vi "AP2x4x ScaleXUnit.vi"(7 "Unit":enum16{"Frequency", "Wavelength"}(ring), 8 "error in":errorcluster, 11 "AP2x4x IN":refnum<visa-resource-name>="TCPIP0::169.254.53.138::5900::SOCKET") -> (0 "error out":errorcluster, 3 "AP2x4x OUT":refnum<visa-resource-name>="TCPIP0::169.254.53.138::5900::SOCKET")   [LabVIEW 2014]
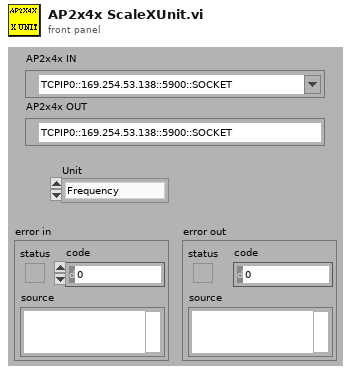
[diagram p1: front panel]
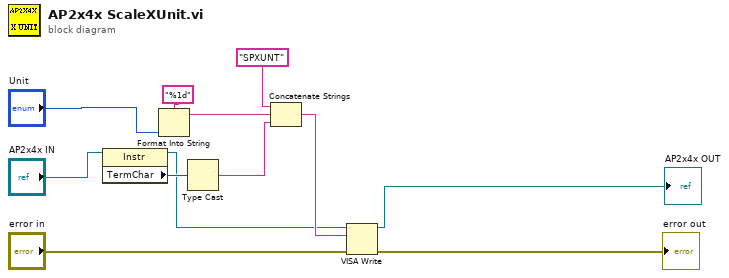
[diagram p0: block diagram]
diagram:
  n1 = property class="Instr"(reference="AP2x4x IN") -> (reference out=w7:refnum<visa-resource-name>, "TermChar"=w10:u8)  [unwired: 1 in, 1 out]
  n2 = Format Into String(format string="%1d", "Unit") -> (resulting string=w5:string)  [unwired: 2 in, 1 out]
  n3 = Type Cast(x=w10) -> (*(type *) &x=w8:string)  [unwired: 1 in]
  n4 = Concatenate Strings("SPXUNT" ("string"), w5, w8) -> (w11:string)
  n5 = VISA Write(VISA resource name=w7, write buffer=w11, error in (no error)="error in") -> (VISA resource name out=→"AP2x4x OUT":refnum<visa-resource-name>, error out=→"error out":errorcluster)  [unwired: 1 out]
